vi "FA_ApplyINItags.vi"(8 "error in (no error)":errorcluster, 11 "INI":T1) -> (0 "error out":errorcluster)   [LabVIEW 2014, in "FA_NativeTypes.lvlib"]
doc: "Uses the INI typdef information to apply changes to INI files"
uses:
  FA_NativeTypes.lvlib
  FA_INI.ctl
  <vilib>/Utility/config.llb/Write Key (String).vi
  <vilib>/Utility/config.llb/NI_LVConfig.lvlib
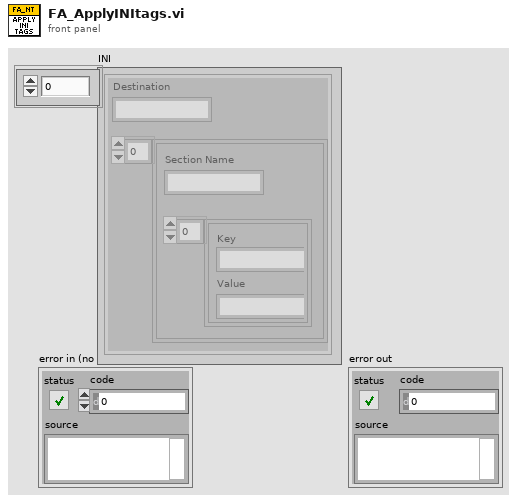
[diagram p1: front panel]
types:
  T1 = typedef "FA_NativeTypes.lvlib/FA_INI.ctl" = cluster{"Destination":string, "Section":cluster{"Section Name":string, "Token":cluster{"Key":string, "Value":string}[]}[]}[]
  T2 = cluster{"Section Name":string, "Token":cluster{"Key":string, "Value":string}[]}[]
  T3 = typedef "NI_LVConfig.lvlib/Config Data RefNum.ctl" = refnum<k1>
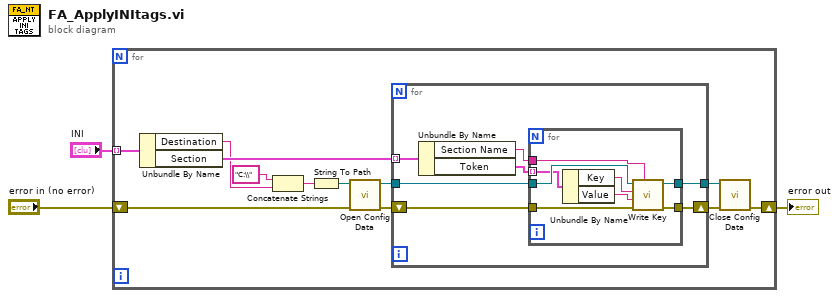
[diagram p0: block diagram]
diagram:
  n1 = for {
    tunnel: "INI" -> [w15] mode=indexing
    shift-right: [w9] -> w3
    shift-left: "error in (no error)" -> [w8]
    n2 = Unbundle By Name(w15) -> ("Destination"=w6:string, "Section"=w14:T2)
    n3 = Concatenate Strings("C:\\" ("string"), w6) -> (w7:string)
    n4 = String To Path(string=w7) -> (path=w13:path)
    n5 = call <vilib>:"Open Config Data.vi"("error in (no error)"=w8, "configuration file path"=w13) -> ("error out"=w11:errorcluster, "refnum"=w12:T3)  [unwired: 7 in, 1 out]
    n6 = for {
      tunnel: w14 -> [w19] mode=indexing
      tunnel: w12 -> [w22]
      shift-right: [w16] -> w10
      shift-left: w11 -> [w21]
      tunnel: [w20] -> w4
      n7 = Unbundle By Name(w19) -> ("Section Name"=w17:string, "Token"=w18:cluster{"Key":string, "Value":string}[])
      n8 = for {
        tunnel: w22 -> [w30]
        tunnel: w21 -> [w29]
        tunnel: [w28] -> w16
        tunnel: [w27] -> w20
        tunnel: w18 -> [w26] mode=indexing
        tunnel: w17 -> [w25]
        n9 = Unbundle By Name(w26) -> ("Key"=w24:string, "Value"=w23:string)
        n10 = call-poly <vilib>:"Write Key.vi"("section"=w25, "error in (no error)"=w29, "value"=w23, "key"=w24, "refnum"=w30) -> ("error out"=w28:errorcluster, "refnum out"=w27:T3)  [unwired: 4 in, 1 out]
      }
    }
    n11 = call <vilib>:"Close Config Data.vi"("error in (no error)"=w10, "refnum"=w4) -> ("error out"=w9:errorcluster)  [unwired: 8 in, 1 out]
  }
  "error out" <- w3
